vi "Brute Force Measurment SubVI Posibly Modded For Trip Prevention System.vi"(8 "error in (no error)":errorcluster, 9 "BoardHandle in":T1, 10 "Stop Program Brute Force":bool, 11 "Barcodes in":string[](array[string])) -> (0 "error out":errorcluster, 1 "BoardHandle out":T1, 2 "Actual Voltage Level (V) 2":dbl format="%#_13g")   [LabVIEW 2020]
panel:
  # "INPUT"
  # "OUTPUT"
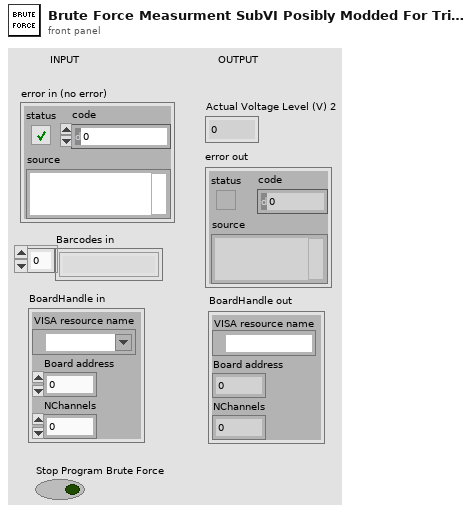
[diagram p1: front panel]
types:
  T1 = cluster{"VISA resource name":refnum<visa-resource-name>, "Board address":u8, "NChannels":u8}
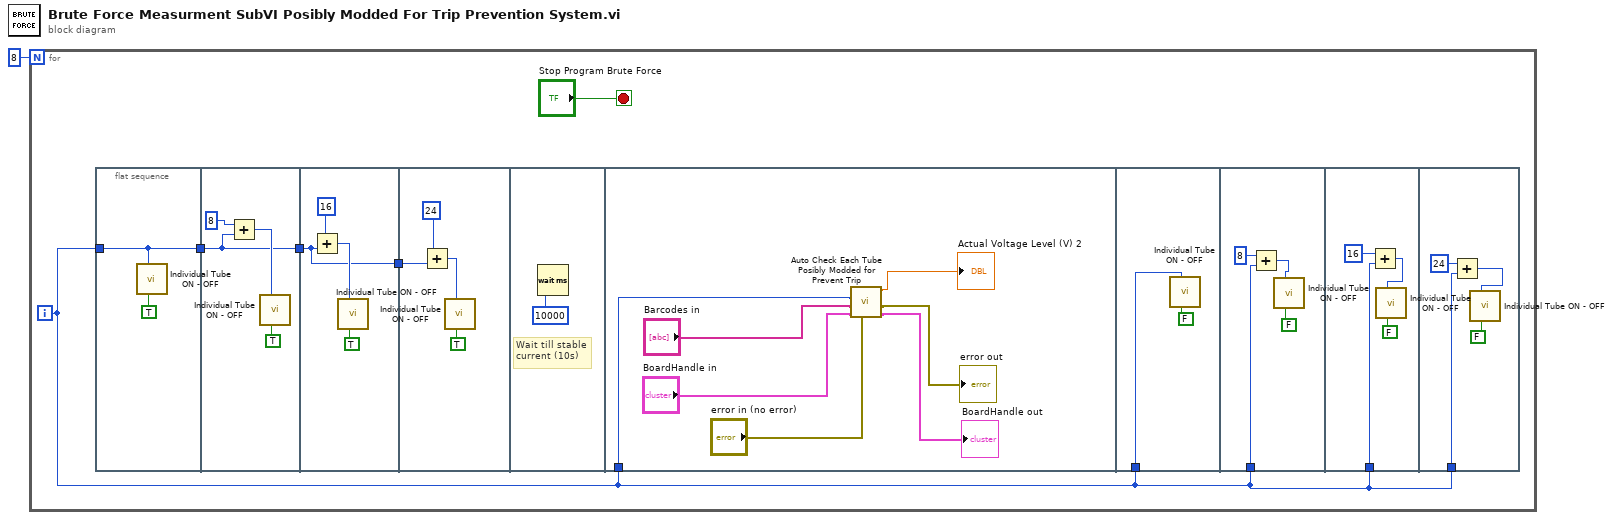
[diagram p0: block diagram]
diagram:
  n1 = for {
    N: 8 -> [_]
    i -> [w2]
    stop <- "Stop Program Brute Force" stop-if-true
    n2 = flat-sequence {
      tunnel: w2 -> [w7]
      tunnel: [w7] -> w5
      tunnel: w5 -> [w10]
      tunnel: [w10] -> w4
      tunnel: w4 -> [w14]
      tunnel: [w14] -> w3
      tunnel: w3 -> [w18]
      tunnel: w2 -> [w25]
      tunnel: w2 -> [w30]
      tunnel: w2 -> [w33]
      tunnel: w2 -> [w37]
      tunnel: w2 -> [w41]
      frame #0 {
        n3 = call "Individual Tube ON - OFF.vi"("Single Tube ON/OFF"=TRUE, "Tube #"=w7) -> ()  [unwired: 10 in]
      }
      frame #1 {
        n4 = Add(x=8, y=w10) -> (x+y=w12:i32)
        n5 = call "Individual Tube ON - OFF.vi"("Single Tube ON/OFF"=TRUE, "Tube #"=w12) -> ()  [unwired: 10 in]
      }
      frame #2 {
        n6 = Add(x=16, y=w14) -> (x+y=w16:i32)
        n7 = call "Individual Tube ON - OFF.vi"("Single Tube ON/OFF"=TRUE, "Tube #"=w16) -> ()  [unwired: 10 in]
      }
      frame #3 {
        n8 = Add(x=24, y=w18) -> (x+y=w20:i32)
        n9 = call "Individual Tube ON - OFF.vi"("Single Tube ON/OFF"=TRUE, "Tube #"=w20) -> ()  [unwired: 10 in]
      }
      frame #4 {
        # "Wait till stable\ncurrent (10s)"
        n10 = Wait (ms)(milliseconds to wait=u32 10000) -> ()  [unwired: 1 out]
      }
      frame #5 {
        n11 = call "Auto Check Each Tube Posibly Modded for Prevent Trip.vi"("error in (no error)"="error in (no error)", "BoardHandle in"="BoardHandle in", "Barcodes in"="Barcodes in", "Tube #"=w25) -> ("BoardHandle out"=→"BoardHandle out":T1, "error out"=→"error out":errorcluster, "Actual Voltage Level (V) 2"=→"Actual Voltage Level (V) 2":dbl)  [unwired: 5 in]
      }
      frame #6 {
        n12 = call "Individual Tube ON - OFF.vi"("Single Tube ON/OFF"=FALSE, "Tube #"=w30) -> ()  [unwired: 10 in]
      }
      frame #7 {
        n13 = Add(x=8, y=w33) -> (x+y=w34:i32)
        n14 = call "Individual Tube ON - OFF.vi"("Single Tube ON/OFF"=FALSE, "Tube #"=w34) -> ()  [unwired: 10 in]
      }
      frame #8 {
        n15 = Add(x=16, y=w37) -> (x+y=w38:i32)
        n16 = call "Individual Tube ON - OFF.vi"("Single Tube ON/OFF"=FALSE, "Tube #"=w38) -> ()  [unwired: 10 in]
      }
      frame #9 {
        n17 = Add(x=24, y=w41) -> (x+y=w42:i32)
        n18 = call "Individual Tube ON - OFF.vi"("Single Tube ON/OFF"=FALSE, "Tube #"=w42) -> ()  [unwired: 10 in]
      }
    }
  }
